vi "AUTON_Index.vi"(0 "Auton Array":dbl[][](array[numeric]), 5 "MeasuredHeading":dbl, 7 "LeftEncoder":dbl, 9 "RightEncoder":dbl) -> (3 "Case":i16, 4 "Right Drive":dbl, 6 "Left Drive":dbl, 8 "Harvester":dbl, 10 "Winch":dbl, 14 "Roller":dbl, 15 "Cam":dbl)   [LabVIEW 2013]
uses:
  Robot Global Data.vi
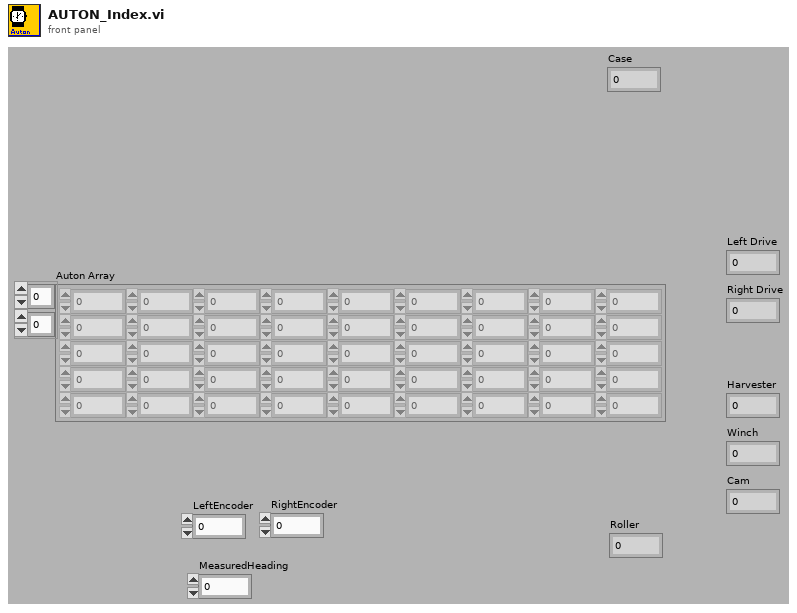
[diagram p1: front panel]
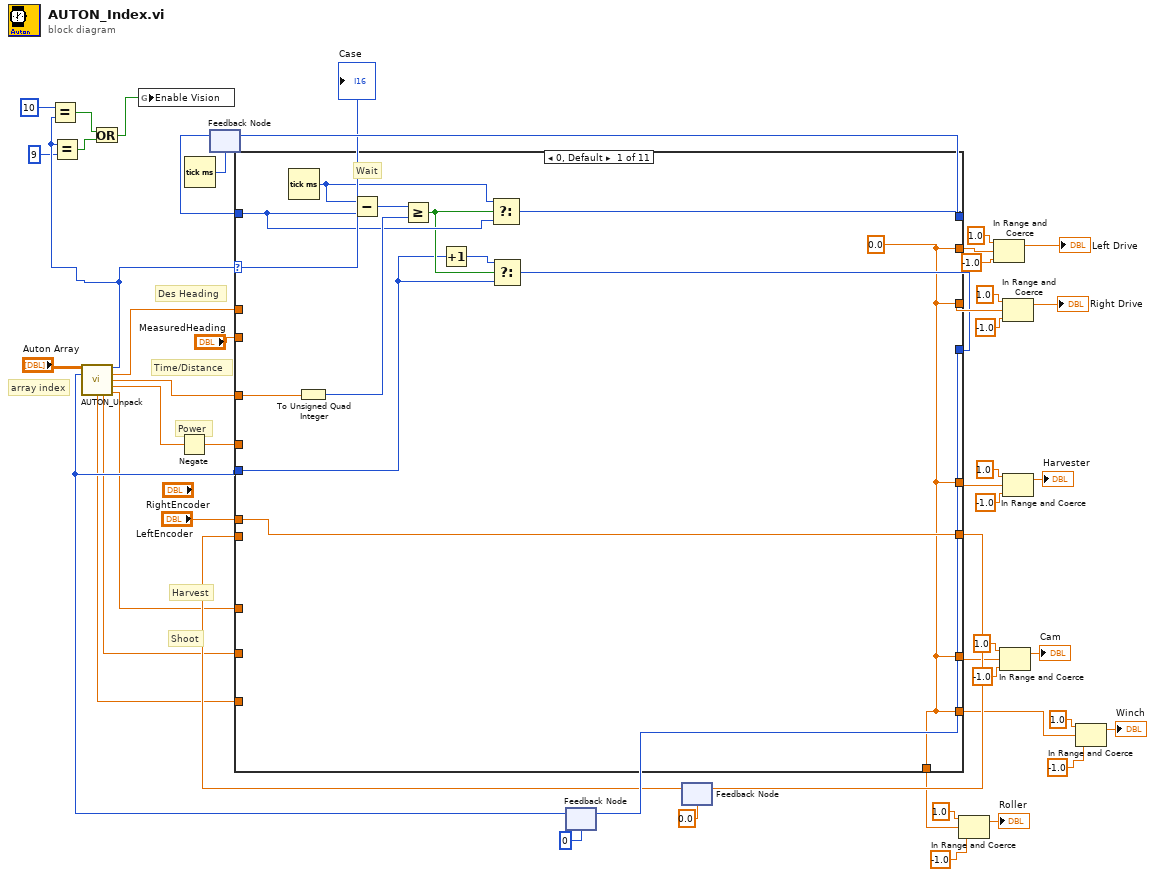
[diagram p0: block diagram]
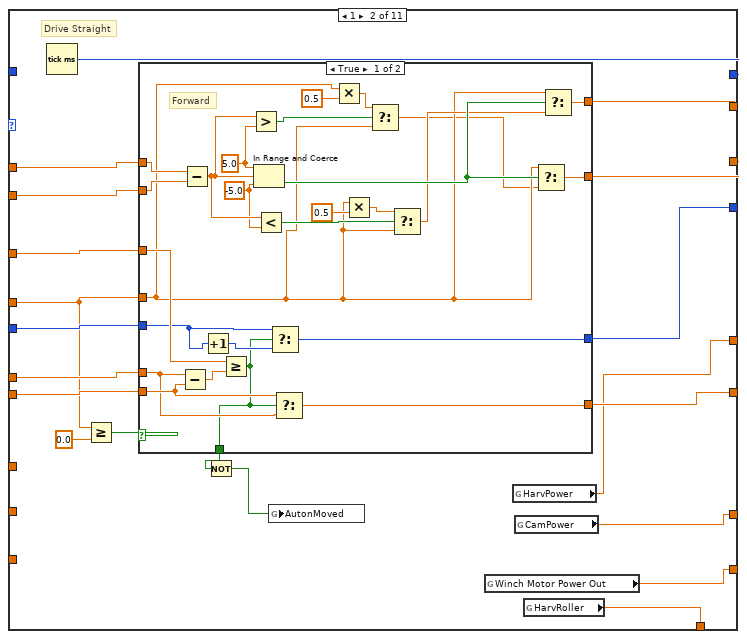
[diagram p2: hidden frame]
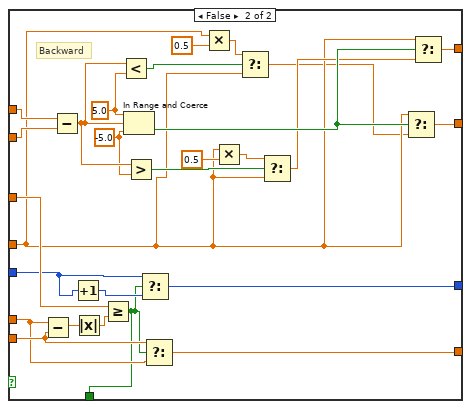
[diagram p3: hidden frame]
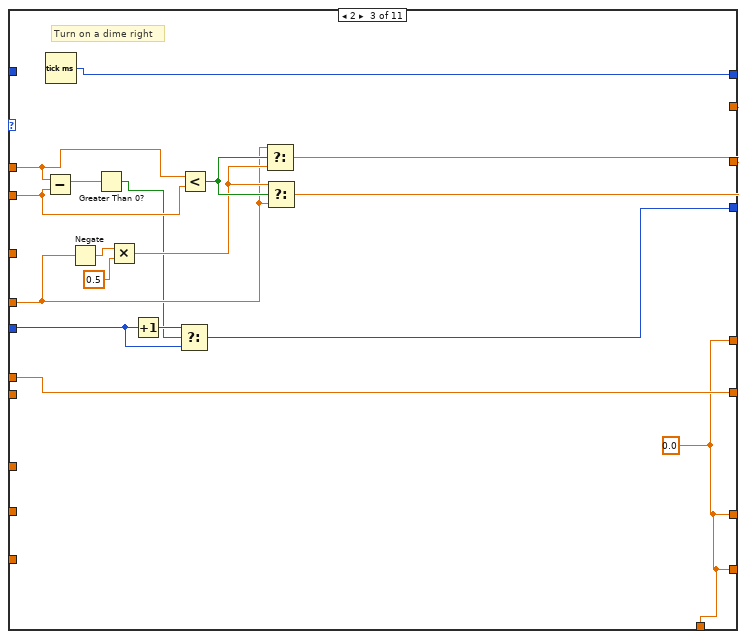
[diagram p4: hidden frame]
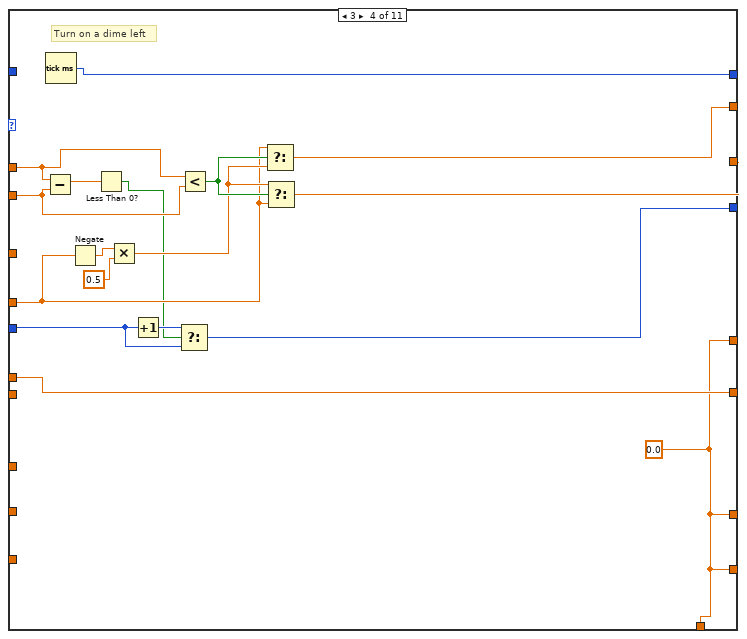
[diagram p5: hidden frame]
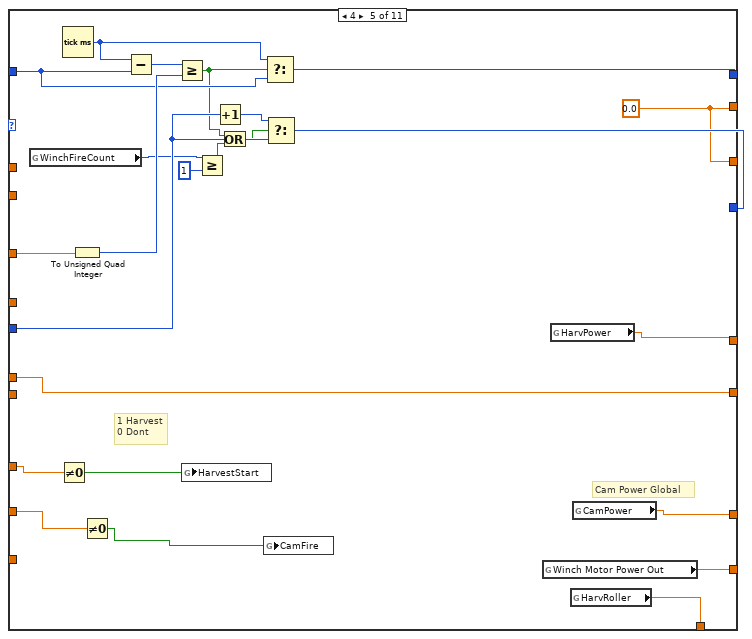
[diagram p6: hidden frame]
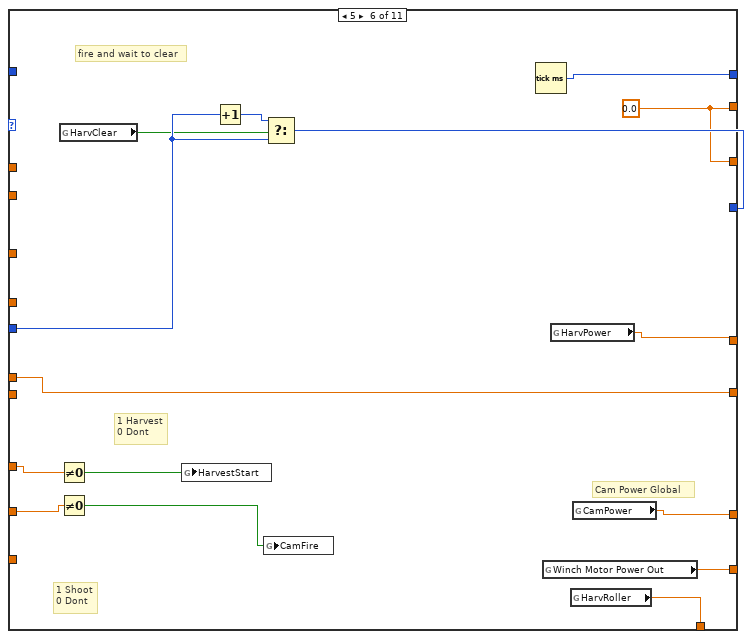
[diagram p7: hidden frame]
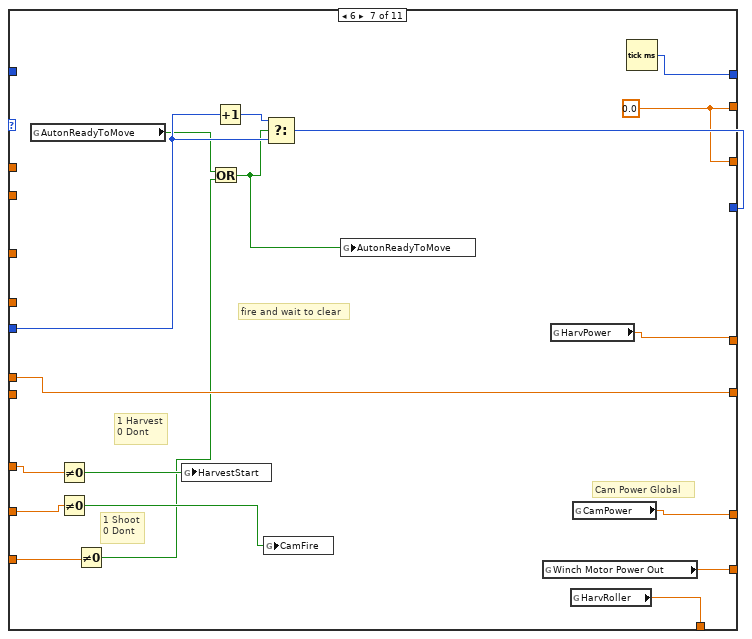
[diagram p8: hidden frame]
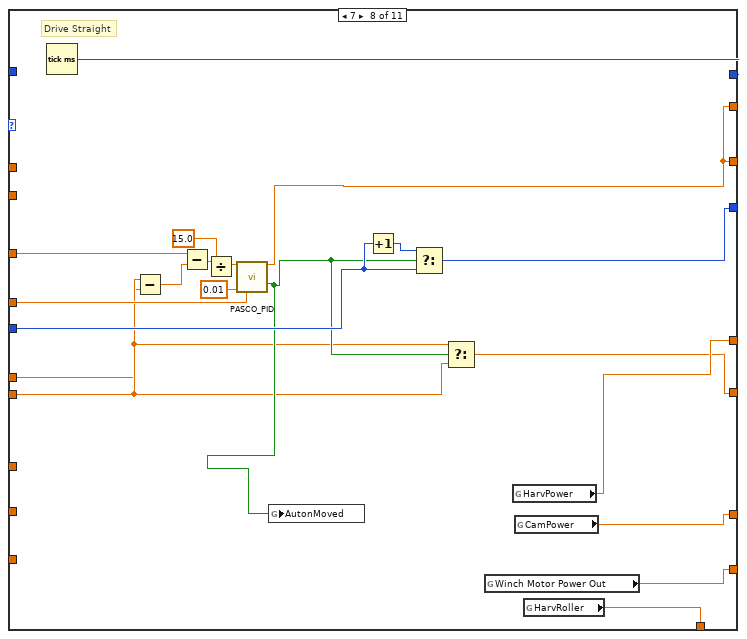
[diagram p9: hidden frame]
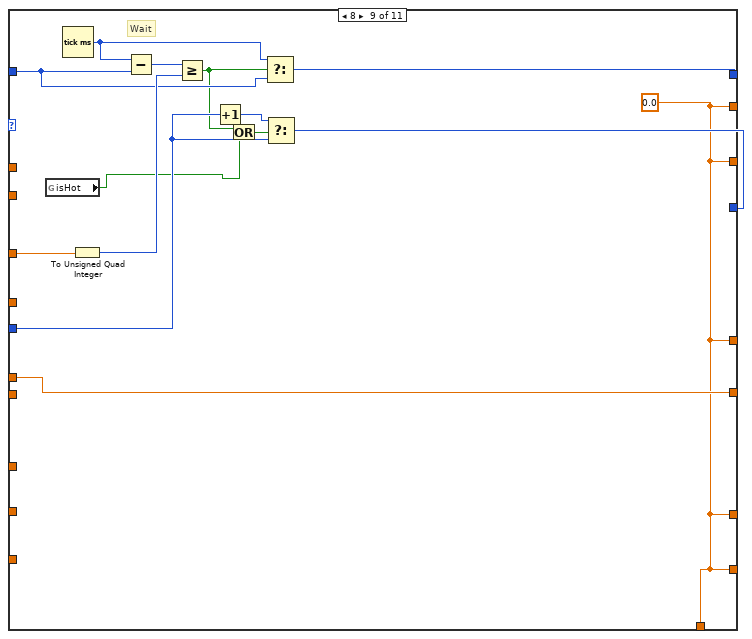
[diagram p10: hidden frame]
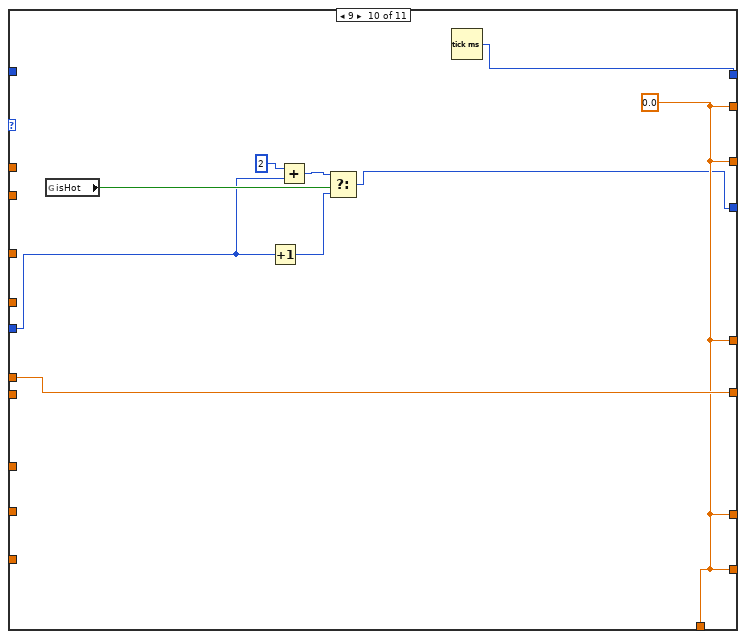
[diagram p11: hidden frame]
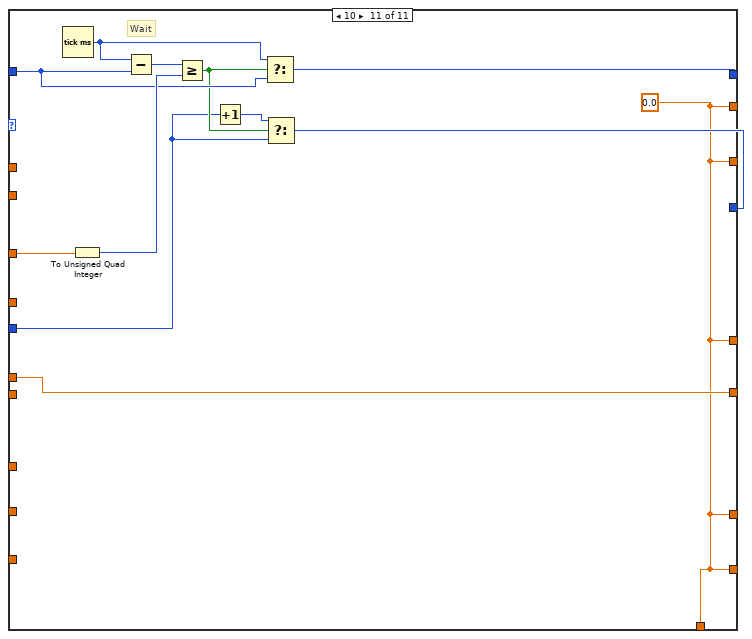
[diagram p12: hidden frame]
diagram:
  # "Shoot"
  # "Harvest"
  # "Des Heading"
  # "Time/Distance"
  # "Power"
  # "array index"
  n1 = Tick Count (ms)() -> (millisecond timer value=w47:u32)
  n2 = feedback #1(w47) -> (w48:u32)
  n3 = feedback #2(0) -> (w29:i32)
  n4 = call "AUTON_Unpack.vi"("all rows"="Auton Array", "Index"=w29) -> ("Primitive ID"=w5:i16, "Desired Heading"=w31:dbl, "Time/Distance"=w30:dbl, "Power"=w17:dbl, "Moved"=w7:dbl, "Shoot"=w14:dbl, "Harvest"=w15:dbl)  [unwired: 7 in]
  "Case" <- w5
  n5 = Equal?(x=i16 10, y=w5) -> (x = y?=w3:bool)
  n6 = Equal?(x=w5, y=i16 9) -> (x = y?=w2:bool)
  n7 = Or(x=w3, y=w2) -> (x .or. y?=w1:bool)
  n8 = global write "Robot Global Data.vi" "Enable Vision"(w1) -> ()
  n9 = Negate(x=w17) -> (-x=w16:dbl)
  n10 = feedback #3(0.0) -> (w33:dbl)
  n11 = case shown="0, Default" w5 {
    tunnel: [w53 w79 w146 w163 w185 w205 w223 w239 w252 w260 w272] -> w35
    tunnel: w29 -> [w54 w74 w149 w166 w186 w206 w224 w237 w253 w262 w273]
    tunnel: [w61 w71 w151 w168 w192 w196 w212 w245 w259 w266 w280] -> w37
    tunnel: w48 -> [w58 _ _ _ w189 _ _ _ w256 _ w277]
    tunnel: w30 -> [w52 w80 _ _ w184 _ _ w229 w251 _ w271]
    tunnel: w31 -> [_ w78 w144 w161 _ _ _ _ _ _ _]
    tunnel: [w50 w76 w147 w164 w183 w204 w222 w227 w249 w267 w269] -> w45
    tunnel: [w50 w75 w148 w165 w183 w204 w222 w227 w249 w267 w269] -> w38
    tunnel: w16 -> [_ w70 w138 w155 _ _ _ w240 _ _ _]
    tunnel: "LeftEncoder" -> [w51 w72 w145 w162 w182 w203 w221 w232 w250 w268 w270]
    tunnel: "MeasuredHeading" -> [_ w77 w143 w160 _ _ _ _ _ _ _]
    tunnel: w33 -> [_ w73 _ _ _ _ _ w233 _ _ _]
    tunnel: [w51 w81 w145 w162 w182 w203 w221 w235 w250 w268 w270] -> w32
    tunnel: [w50 w67 w135 w152 w180 w201 w219 w244 w249 w267 w269] -> w19
    tunnel: [w50 w65 w135 w152 w181 w202 w220 w242 w249 w267 w269] -> w18
    tunnel: w15 -> [_ _ _ _ w177 w199 w217 _ _ _ _]
    tunnel: w14 -> [_ _ _ _ w179 w194 w214 _ _ _ _]
    tunnel: [w50 w66 w135 w152 w178 w200 w218 w243 w249 w267 w269] -> w13
    tunnel: [w50 w64 w135 w152 w174 w197 w215 w241 w249 w267 w269] -> w9
    tunnel: w7 -> [_ _ _ _ _ _ w211 _ _ _ _]
    frame 0, Default {
      w50 = 0.0 ("Numeric")
      # "Wait"
      n12 = Tick Count (ms)() -> (millisecond timer value=w57:u32)
      n13 = To Unsigned Quad Integer(1:w52) -> (0:w59:u64)
      n14 = Subtract(x=w57, y=w58) -> (x-y=w60:u32)
      n15 = Greater Or Equal?(x=w60, y=w59) -> (x >= y?=w56:bool)
      n16 = Increment(x=w54) -> (x+1=w55:i32)
      n17 = Select(t=w57, s=w56, f=w58) -> (s? t:f=w61:u32)
      n18 = Select(t=w55, s=w56, f=w54) -> (s? t:f=w53:i32)
    }
    frame 1 {
      # "Drive Straight"
      n19 = Tick Count (ms)() -> (millisecond timer value=w71:u32)
      n20 = Greater Or Equal?(x=w70, y=0.0) -> (x >= y?=w68:bool)
      n21 = case shown="True" w68 {
        tunnel: [w107 w134] -> w81
        tunnel: w80 -> [w105 w133]
        tunnel: [w104 w132] -> w79
        tunnel: w78 -> [w103 w131]
        tunnel: w77 -> [w102 w130]
        tunnel: [w100 w128] -> w76
        tunnel: [w99 w127] -> w75
        tunnel: w70 -> [w88 w116]
        tunnel: w74 -> [w85 w113]
        tunnel: w73 -> [w84 w112]
        tunnel: w72 -> [w83 w111]
        tunnel: [w82 w108] -> w63
        frame True {
          w96 = -5.0 ("lower limit")
          w98 = 5.0 ("upper limit")
          # "Forward"
          n22 = Subtract(x=w83, y=w84) -> (x-y=w106:dbl)
          n23 = Subtract(x=w103, y=w102) -> (x-y=w97:dbl)
          n24 = Increment(x=w85) -> (x+1=w86:i32)
          n25 = Greater Or Equal?(x=w105, y=w106) -> (x >= y?=w82:bool)
          n26 = Greater?(x=w97, y=w98) -> (0:w91:bool)
          n27 = In Range and Coerce(upper limit=w98, x=w97, lower limit=w96) -> (In Range?=w101:bool)  [unwired: 1 out]
          n28 = Less?(x=w97, y=w96) -> (x < y?=w95:bool)
          n29 = Select(t=w85, s=w82, f=w86) -> (s? t:f=w104:i32)
          n30 = Select(t=w84, s=w82, f=w83) -> (s? t:f=w107:dbl)
          n31 = Multiply(x=w88, y=0.5) -> (x*y=w90:dbl)
          n32 = Multiply(x=w88, y=0.5) -> (x*y=w93:dbl)
          n33 = Select(t=w90, s=w91, f=w88) -> (s? t:f=w87:dbl)
          n34 = Select(t=w93, s=w95, f=w88) -> (s? t:f=w92:dbl)
          n35 = Select(t=w88, s=w101, f=w87) -> (s? t:f=w99:dbl)
          n36 = Select(t=w88, s=w101, f=w92) -> (s? t:f=w100:dbl)
        }
        frame False {
          w124 = -5.0 ("lower limit")
          w126 = 5.0 ("upper limit")
          # "Backward"
          n37 = Subtract(x=w111, y=w112) -> (x-y=w109:dbl)
          n38 = Subtract(x=w131, y=w130) -> (x-y=w125:dbl)
          n39 = Increment(x=w113) -> (x+1=w114:i32)
          n40 = Absolute Value(x=w109) -> (abs(x)=w110:dbl)
          n41 = Greater Or Equal?(x=w133, y=w110) -> (x >= y?=w108:bool)
          n42 = Less?(x=w125, y=w126) -> (x < y?=w119:bool)
          n43 = In Range and Coerce(upper limit=w126, x=w125, lower limit=w124) -> (In Range?=w129:bool)  [unwired: 1 out]
          n44 = Greater?(x=w125, y=w124) -> (0:w123:bool)
          n45 = Select(t=w113, s=w108, f=w114) -> (s? t:f=w132:i32)
          n46 = Select(t=w112, s=w108, f=w111) -> (s? t:f=w134:dbl)
          n47 = Multiply(x=w116, y=0.5) -> (x*y=w118:dbl)
          n48 = Multiply(x=w116, y=0.5) -> (x*y=w121:dbl)
          n49 = Select(t=w118, s=w119, f=w116) -> (s? t:f=w115:dbl)
          n50 = Select(t=w121, s=w123, f=w116) -> (s? t:f=w120:dbl)
          n51 = Select(t=w116, s=w129, f=w115) -> (s? t:f=w127:dbl)
          n52 = Select(t=w116, s=w129, f=w120) -> (s? t:f=w128:dbl)
        }
      }
      n53 = Not(x=w63) -> (.not. x?=w62:bool)
      n54 = global write "Robot Global Data.vi" "AutonMoved"(w62) -> ()
      n55 = global read "Robot Global Data.vi" "Winch Motor Power Out"() -> (w66:dbl)
      n56 = global read "Robot Global Data.vi" "HarvPower"() -> (w65:dbl)
      n57 = global read "Robot Global Data.vi" "CamPower"() -> (w67:dbl)
      n58 = global read "Robot Global Data.vi" "HarvRoller"() -> (w64:dbl)
    }
    frame 2 {
      w135 = 0.0 ("Numeric")
      # "Turn on a dime right"
      n59 = Subtract(x=w144, y=w143) -> (x-y=w137:dbl)
      n60 = Tick Count (ms)() -> (millisecond timer value=w151:u32)
      n61 = Negate(x=w138) -> (-x=w141:dbl)
      n62 = Greater Than 0?(x=w137) -> (x > 0?=w136:bool)
      n63 = Multiply(x=w141, y=0.5) -> (x*y=w139:dbl)
      n64 = Increment(x=w149) -> (x+1=w150:i32)
      n65 = Select(t=w150, s=w136, f=w149) -> (s? t:f=w146:i32)
      n66 = Less?(x=w144, y=w143) -> (x < y?=w142:bool)
      n67 = Select(t=w138, s=w142, f=w139) -> (s? t:f=w147:dbl)
      n68 = Select(t=w139, s=w142, f=w138) -> (s? t:f=w148:dbl)
    }
    frame 3 {
      w152 = 0.0 ("Numeric")
      # "Turn on a dime left"
      n69 = Subtract(x=w161, y=w160) -> (x-y=w154:dbl)
      n70 = Tick Count (ms)() -> (millisecond timer value=w168:u32)
      n71 = Negate(x=w155) -> (-x=w158:dbl)
      n72 = Less Than 0?(x=w154) -> (x < 0?=w153:bool)
      n73 = Multiply(x=w158, y=0.5) -> (x*y=w156:dbl)
      n74 = Increment(x=w166) -> (x+1=w167:i32)
      n75 = Select(t=w167, s=w153, f=w166) -> (s? t:f=w163:i32)
      n76 = Less?(x=w161, y=w160) -> (x < y?=w159:bool)
      n77 = Select(t=w155, s=w159, f=w156) -> (s? t:f=w164:dbl)
      n78 = Select(t=w156, s=w159, f=w155) -> (s? t:f=w165:dbl)
    }
    frame 4 {
      w183 = 0.0 ("Numeric")
      # "1 Harvest\n0 Dont"
      # "Cam Power Global"
      n79 = global read "Robot Global Data.vi" "WinchFireCount"() -> (w170:i32)
      n80 = Not Equal To 0?(x=w177) -> (x != 0?=w176:bool)
      n81 = Tick Count (ms)() -> (millisecond timer value=w188:u32)
      n82 = To Unsigned Quad Integer(1:w184) -> (0:w190:u64)
      n83 = Not Equal To 0?(x=w179) -> (x != 0?=w175:bool)
      n84 = Subtract(x=w188, y=w189) -> (x-y=w191:u32)
      n85 = Greater Or Equal?(x=w191, y=w190) -> (x >= y?=w172:bool)
      n86 = global write "Robot Global Data.vi" "HarvestStart"(w176) -> ()
      n87 = Greater Or Equal?(x=w170, y=1) -> (x >= y?=w171:bool)
      n88 = Increment(x=w186) -> (x+1=w187:i32)
      n89 = Or(x=w172, y=w171) -> (x .or. y?=w173:bool)
      n90 = global write "Robot Global Data.vi" "CamFire"(w175) -> ()
      n91 = Select(t=w188, s=w172, f=w189) -> (s? t:f=w192:u32)
      n92 = Select(t=w187, s=w173, f=w186) -> (s? t:f=w185:i32)
      n93 = global read "Robot Global Data.vi" "Winch Motor Power Out"() -> (w178:dbl)
      n94 = global read "Robot Global Data.vi" "HarvPower"() -> (w181:dbl)
      n95 = global read "Robot Global Data.vi" "HarvRoller"() -> (w174:dbl)
      n96 = global read "Robot Global Data.vi" "CamPower"() -> (w180:dbl)
    }
    frame 5 {
      w204 = 0.0 ("Numeric")
      # "fire and wait to clear"
      # "1 Harvest\n0 Dont"
      # "1 Shoot\n0 Dont"
      # "Cam Power Global"
      n97 = Not Equal To 0?(x=w199) -> (x != 0?=w198:bool)
      n98 = Not Equal To 0?(x=w194) -> (x != 0?=w193:bool)
      n99 = global read "Robot Global Data.vi" "HarvClear"() -> (w195:bool)
      n100 = global write "Robot Global Data.vi" "HarvestStart"(w198) -> ()
      n101 = Increment(x=w206) -> (x+1=w207:i32)
      n102 = global write "Robot Global Data.vi" "CamFire"(w193) -> ()
      n103 = Select(t=w207, s=w195, f=w206) -> (s? t:f=w205:i32)
      n104 = Tick Count (ms)() -> (millisecond timer value=w196:u32)
      n105 = global read "Robot Global Data.vi" "Winch Motor Power Out"() -> (w200:dbl)
      n106 = global read "Robot Global Data.vi" "HarvPower"() -> (w202:dbl)
      n107 = global read "Robot Global Data.vi" "HarvRoller"() -> (w197:dbl)
      n108 = global read "Robot Global Data.vi" "CamPower"() -> (w201:dbl)
    }
    frame 6 {
      w222 = 0.0 ("Numeric")
      # "fire and wait to clear"
      # "1 Harvest\n0 Dont"
      # "1 Shoot\n0 Dont"
      # "Cam Power Global"
      n109 = global read "Robot Global Data.vi" "AutonReadyToMove"() -> (w209:bool)
      n110 = Not Equal To 0?(x=w217) -> (x != 0?=w216:bool)
      n111 = Not Equal To 0?(x=w214) -> (x != 0?=w213:bool)
      n112 = Not Equal To 0?(x=w211) -> (x != 0?=w210:bool)
      n113 = global write "Robot Global Data.vi" "HarvestStart"(w216) -> ()
      n114 = Or(x=w209, y=w210) -> (x .or. y?=w208:bool)
      n115 = Increment(x=w224) -> (x+1=w225:i32)
      n116 = global write "Robot Global Data.vi" "CamFire"(w213) -> ()
      n117 = Select(t=w225, s=w208, f=w224) -> (s? t:f=w223:i32)
      n118 = global write "Robot Global Data.vi" "AutonReadyToMove"(w208) -> ()
      n119 = global read "Robot Global Data.vi" "Winch Motor Power Out"() -> (w218:dbl)
      n120 = global read "Robot Global Data.vi" "HarvPower"() -> (w220:dbl)
      n121 = global read "Robot Global Data.vi" "HarvRoller"() -> (w215:dbl)
      n122 = global read "Robot Global Data.vi" "CamPower"() -> (w219:dbl)
      n123 = Tick Count (ms)() -> (millisecond timer value=w212:u32)
    }
    frame 7 {
      # "Drive Straight"
      n124 = Tick Count (ms)() -> (millisecond timer value=w245:u32)
      n125 = Subtract(x=w233, y=w232) -> (x-y=w234:dbl)
      n126 = Subtract(x=w229, y=w234) -> (x-y=w230:dbl)
      n127 = Divide(x=w230, y=15.0) -> (x/y=w231:dbl)
      n128 = call "PASCO_PID.vi"("Delta"=w231, "Deadband"=0.01, "P Gain"=w240) -> ("Output"=w227:dbl, "IsThere"=w236:bool)  [unwired: 11 in]
      n129 = global write "Robot Global Data.vi" "AutonMoved"(w236) -> ()
      n130 = Increment(x=w237) -> (x+1=w238:i32)
      n131 = Select(t=w238, s=w236, f=w237) -> (s? t:f=w239:i32)
      n132 = Select(t=w232, s=w236, f=w233) -> (s? t:f=w235:dbl)
      n133 = global read "Robot Global Data.vi" "Winch Motor Power Out"() -> (w243:dbl)
      n134 = global read "Robot Global Data.vi" "HarvPower"() -> (w242:dbl)
      n135 = global read "Robot Global Data.vi" "CamPower"() -> (w244:dbl)
      n136 = global read "Robot Global Data.vi" "HarvRoller"() -> (w241:dbl)
    }
    frame 8 {
      w249 = 0.0 ("Numeric")
      # "Wait"
      n137 = global read "Robot Global Data.vi" "isHot"() -> (w246:bool)
      n138 = Tick Count (ms)() -> (millisecond timer value=w255:u32)
      n139 = To Unsigned Quad Integer(1:w251) -> (0:w257:u64)
      n140 = Subtract(x=w255, y=w256) -> (x-y=w258:u32)
      n141 = Greater Or Equal?(x=w258, y=w257) -> (x >= y?=w248:bool)
      n142 = Increment(x=w253) -> (x+1=w254:i32)
      n143 = Or(x=w248, y=w246) -> (x .or. y?=w247:bool)
      n144 = Select(t=w255, s=w248, f=w256) -> (s? t:f=w259:u32)
      n145 = Select(t=w254, s=w247, f=w253) -> (s? t:f=w252:i32)
    }
    frame 9 {
      w267 = 0.0 ("Numeric")
      n146 = global read "Robot Global Data.vi" "isHot"() -> (w264:bool)
      n147 = Increment(x=w262) -> (x+1=w265:i32)
      n148 = Add(x=2, y=w262) -> (x+y=w263:i32)
      n149 = Select(t=w263, s=w264, f=w265) -> (s? t:f=w260:i32)
      n150 = Tick Count (ms)() -> (millisecond timer value=w266:u32)
    }
    frame 10 {
      w269 = 0.0 ("Numeric")
      # "Wait"
      n151 = Tick Count (ms)() -> (millisecond timer value=w276:u32)
      n152 = To Unsigned Quad Integer(1:w271) -> (0:w278:u64)
      n153 = Subtract(x=w276, y=w277) -> (x-y=w279:u32)
      n154 = Greater Or Equal?(x=w279, y=w278) -> (x >= y?=w275:bool)
      n155 = Increment(x=w273) -> (x+1=w274:i32)
      n156 = Select(t=w276, s=w275, f=w277) -> (s? t:f=w280:u32)
      n157 = Select(t=w274, s=w275, f=w273) -> (s? t:f=w272:i32)
    }
  }
  n158 = feedback-in #1(w37) -> ()
  n159 = feedback-in #2(w35) -> ()
  n160 = feedback-in #3(w32) -> ()
  n161 = In Range and Coerce(upper limit=1.0, x=w9, lower limit=-1.0) -> (coerced(x)=→"Roller":dbl)  [unwired: 1 out]
  n162 = In Range and Coerce(upper limit=1.0, x=w45, lower limit=-1.0) -> (coerced(x)=→"Left Drive":dbl)  [unwired: 1 out]
  n163 = In Range and Coerce(upper limit=1.0, x=w19, lower limit=-1.0) -> (coerced(x)=→"Cam":dbl)  [unwired: 1 out]
  n164 = In Range and Coerce(upper limit=1.0, x=w38, lower limit=-1.0) -> (coerced(x)=→"Right Drive":dbl)  [unwired: 1 out]
  n165 = In Range and Coerce(upper limit=1.0, x=w18, lower limit=-1.0) -> (coerced(x)=→"Harvester":dbl)  [unwired: 1 out]
  n166 = In Range and Coerce(upper limit=1.0, x=w13, lower limit=-1.0) -> (coerced(x)=→"Winch":dbl)  [unwired: 1 out]
